vi "TestVI.vi"() -> ()   [LabVIEW 2015, in "BT-Android_interface.lvlib"]
uses:
  BT-Android_interface.lvlib
panel:
  in  "停止":bool
  out "波形图表":u8[](graph)
  out "timeout?":bool
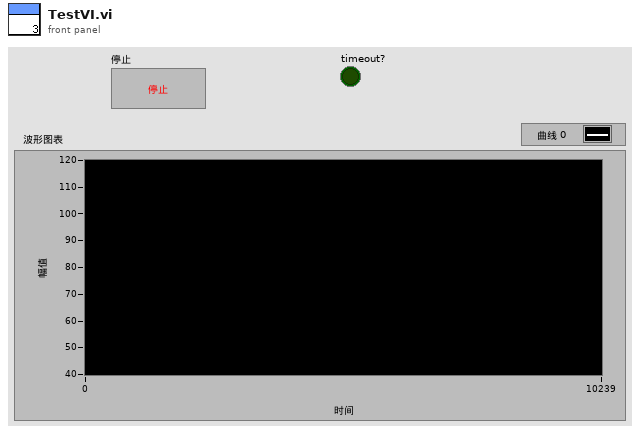
[diagram p1: front panel]
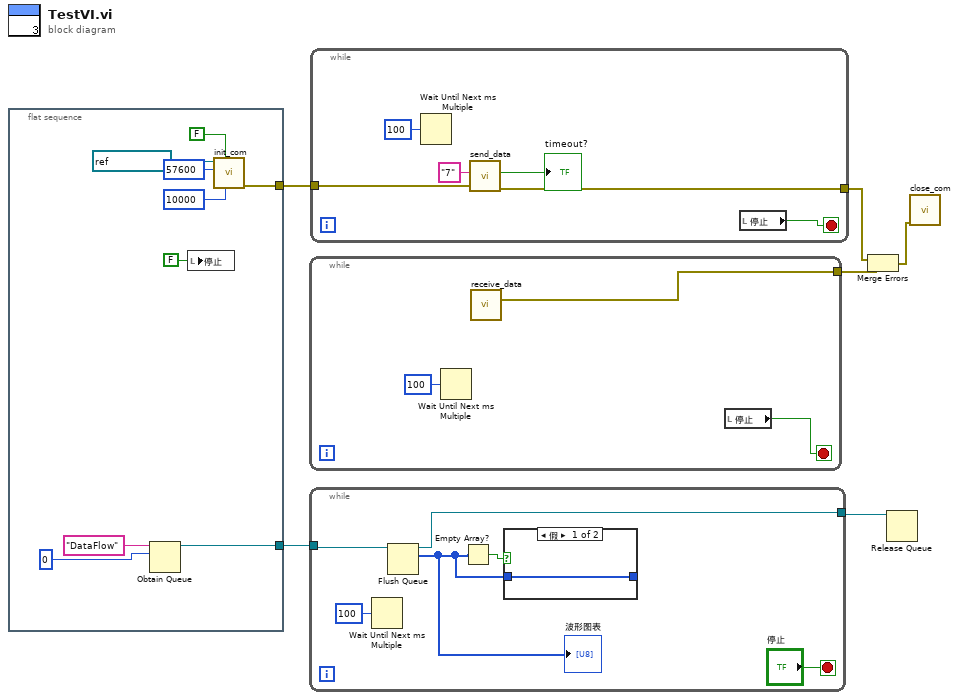
[diagram p0: block diagram]
diagram:
  n1 = flat-sequence {
    tunnel: [w15] -> w6
    tunnel: [w10] -> w2
    frame #0 {
      n2 = Obtain Queue(name (unnamed)="DataFlow", element data type=u8 0) -> (queue out=w10:refnum<queue>)  [unwired: 3 in, 2 out]
      n3 = local write "停止"(FALSE ("停止")) -> ()
      n4 = call "init_com.vi"("timeout (10sec)"=u32 10000, "End Write on Termination Character?"=FALSE, "port"=u32 57600, "VISA resource name"=refnum<visa-resource-name> "127.0.0.1") -> ("error out"=w15:errorcluster)  [unwired: 7 in]
    }
  }
  n5 = while {
    tunnel: [w18] -> w4
    stop <- w16 stop-if-true
    n6 = Wait Until Next ms Multiple(millisecond multiple=u32 100 ("毫秒倍数")) -> ()  [unwired: 1 out]
    n7 = call "receive_data.vi"() -> ("error out"=w18:errorcluster)  [unwired: 14 in, 1 out]
    n8 = local read "停止"() -> (w16:bool)
  }
  n9 = while {
    tunnel: w2 -> [w24]
    tunnel: [w23] -> w1
    stop <- "停止" stop-if-true
    n10 = Wait Until Next ms Multiple(millisecond multiple=u32 100 ("毫秒倍数")) -> ()  [unwired: 1 out]
    n11 = Flush Queue(queue=w24) -> (queue out=w23:refnum<queue>, remaining elements=w19:u8[])  [unwired: 1 in, 1 out]
    "波形图表" <- w19
    n12 = Empty Array?(array=w19) -> (empty?=w20:bool)
    n13 = case shown="假" w20 {
      tunnel: w19 -> [w25 _]
      tunnel: [w25 _] -> _
      frame False {
      }
      frame True {
      }
    }
  }
  n14 = while {
    tunnel: w6 -> [w31]
    tunnel: [w30] -> w5
    stop <- w26 stop-if-true
    n15 = Wait Until Next ms Multiple(millisecond multiple=u32 100 ("毫秒倍数")) -> ()  [unwired: 1 out]
    n16 = call "send_data.vi"("error in (no error)"=w31, "send data (string)"="7") -> ("error out"=w30:errorcluster, "timeout?"=→"timeout?":bool)  [unwired: 8 in]
    n17 = local read "停止"() -> (w26:bool)
  }
  n18 = Merge Errors(w5, w4) -> (w3:errorcluster)
  n19 = Release Queue(queue=w1) -> ()  [unwired: 2 in, 3 out]
  n20 = call "close_com.vi"("error in (no error)"=w3) -> ()  [unwired: 10 in, 1 out]
